vi "CalcData.vi"(8 "error in (no error)":errorcluster, 10 "Complex Data (in)":csg[](array[numeric])) -> (0 "error out":errorcluster, 2 "Array out":csg[](array[numeric]))   [LabVIEW 2014]
uses:
  GlobalVariables.vi
  <vilib>/rvi/interface/RandomDataEmulation/nirviRandomDataDMAMethods.vi
  <vilib>/rvi/interface/nirviMethod/nirviMethod.xnode
  Fpga-Version/PXI-7953R/Fft.vi
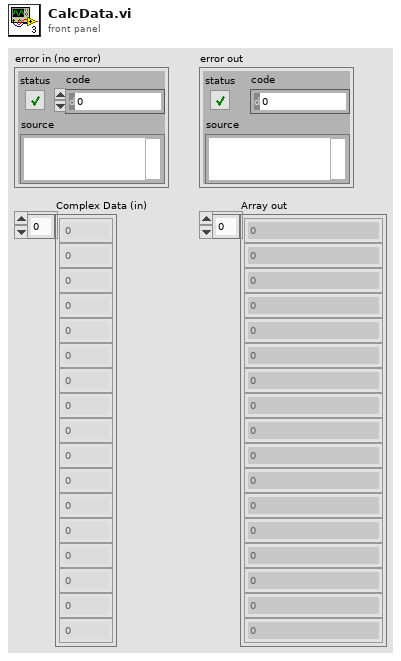
[diagram p1: front panel]
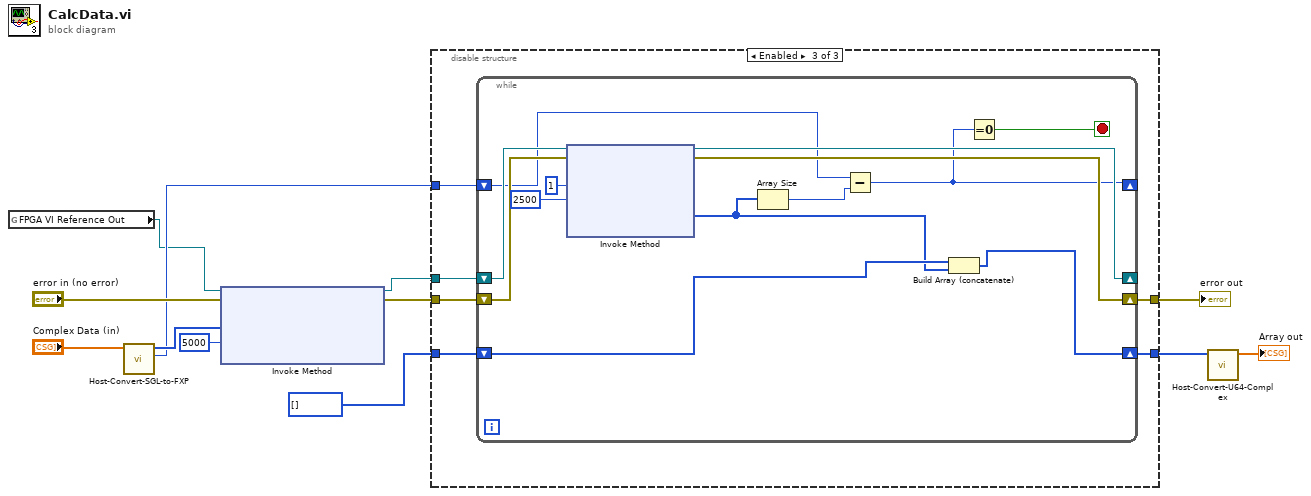
[diagram p0: block diagram]
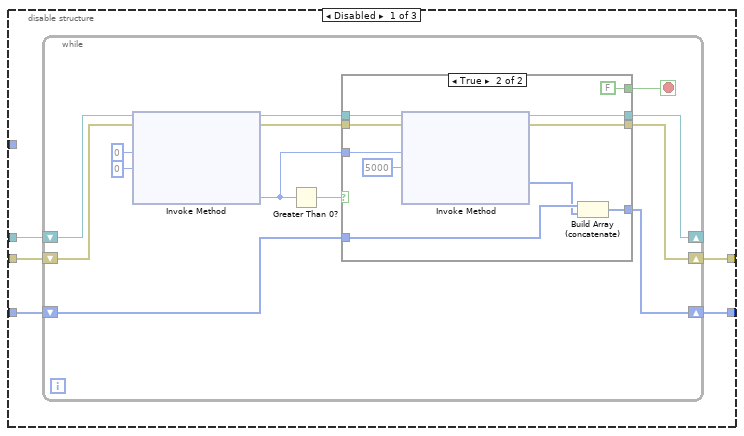
[diagram p2: hidden frame]
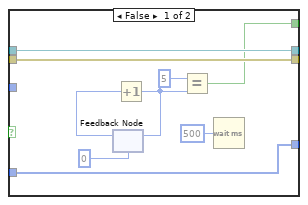
[diagram p3: hidden frame]
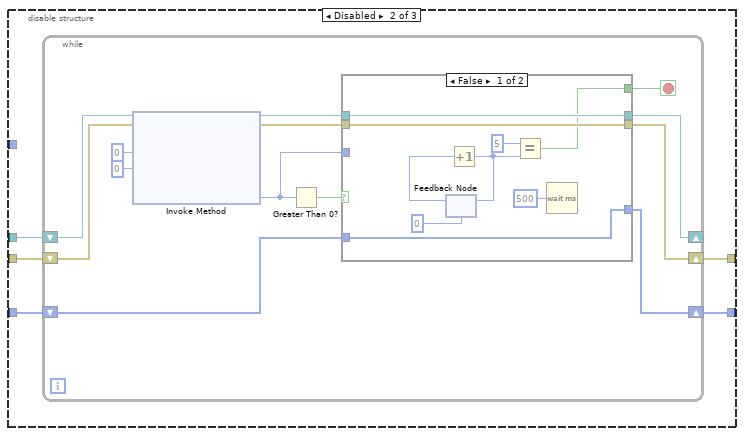
[diagram p4: hidden frame]
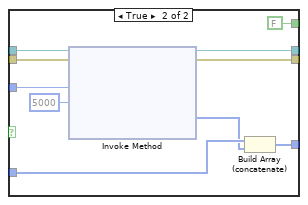
[diagram p5: hidden frame]
diagram:
  n1 = global read "GlobalVariables.vi" "FPGA VI Reference Out"() -> (w2:refnum<k20>)
  n2 = call "Host-Convert-SGL-to-FXP.vi"("Complex Data (in)"="Complex Data (in)") -> ("[FPGA] Array Size"=w3:u64, "Complex Data Ready for FPGA (out)"=w12:u64[])  [unwired: 9 in]
  n3 = xnode "Invoke Method"("FPGA VI Reference In"=w2, "error in"="error in (no error)", "Data"=w12, "Timeout (ms)"=5000) -> ("FPGA VI Reference Out"=w6:refnum<k20>, "error out"=w7:errorcluster)  [unwired: 1 out]
  n4 = disable-structure shown="Enabled" {
    disable-tunnel: [w17 w54 w88] -> w10
    disable-tunnel: u64[] [] -> [w16 w53 w90]
    disable-tunnel: [w15 w52 w89] -> w8
    disable-tunnel: w7 -> [w14 w51 w91]
    disable-tunnel: w6 -> [w13 w50 w92]
    disable-tunnel: w3 -> [_ _ w87]
    frame Disabled {
      n5 = while {
        shift-right: [w19] -> _
        shift-left: w13 -> [w30]
        shift-right: [w20] -> w15
        shift-left: w14 -> [w21]
        shift-right: [w24] -> w17
        shift-left: w16 -> [w23]
        stop <- w18 stop-if-true
        n6 = xnode "Invoke Method"("FPGA VI Reference In"=w30, "error in"=w21, "Number of Elements"=u32 0, "Timeout (ms)"=0) -> ("FPGA VI Reference Out"=w26:refnum<k20>, "error out"=w22:errorcluster, "Elements Remaining"=w25:u32)  [unwired: 1 out]
        n7 = Greater Than 0?(x=w25) -> (x > 0?=w27:bool)
        n8 = case shown="True" w27 {
          tunnel: w26 -> [w37 w49]
          tunnel: w25 -> [_ w48]
          tunnel: [w39 w44] -> w24
          tunnel: w23 -> [w39 w46]
          tunnel: w22 -> [w38 w43]
          tunnel: [w38 w42] -> w20
          tunnel: [w37 w41] -> w19
          tunnel: [w32 FALSE] -> w18
          frame False {
            n9 = feedback #1(0) -> (w35:i32)
            n10 = Increment(x=w35) -> (x+1=w34:i32)
            n11 = feedback-in #1(w34) -> ()
            n12 = Equal?(x=5, y=w34) -> (x = y?=w32:bool)
            n13 = Wait (ms)(milliseconds to wait=u32 500) -> ()  [unwired: 1 out]
          }
          frame True {
            n14 = xnode "Invoke Method"("FPGA VI Reference In"=w49, "error in"=w43, "Number of Elements"=w48, "Timeout (ms)"=5000) -> ("FPGA VI Reference Out"=w41:refnum<k20>, "error out"=w42:errorcluster, "Data"=w45:u64[])  [unwired: 1 out]
            n15 = Build Array (concatenate)(w46, w45) -> (w44:u64[])
          }
        }
      }
    }
    frame Disabled {
      n16 = while {
        shift-right: [w56] -> _
        shift-left: w50 -> [w67]
        shift-right: [w57] -> w52
        shift-left: w51 -> [w58]
        shift-right: [w61] -> w54
        shift-left: w53 -> [w60]
        stop <- w55 stop-if-true
        n17 = xnode "Invoke Method"("FPGA VI Reference In"=w67, "error in"=w58, "Number of Elements"=u32 0, "Timeout (ms)"=0) -> ("FPGA VI Reference Out"=w63:refnum<k20>, "error out"=w59:errorcluster, "Elements Remaining"=w62:u32)  [unwired: 1 out]
        n18 = Greater Than 0?(x=w62) -> (x > 0?=w64:bool)
        n19 = case shown="False" w64 {
          tunnel: w63 -> [w74 w86]
          tunnel: w62 -> [_ w85]
          tunnel: [w76 w81] -> w61
          tunnel: w60 -> [w76 w83]
          tunnel: w59 -> [w75 w80]
          tunnel: [w75 w79] -> w57
          tunnel: [w74 w78] -> w56
          tunnel: [w69 FALSE] -> w55
          frame False {
            n20 = feedback #2(0) -> (w72:i32)
            n21 = Increment(x=w72) -> (x+1=w71:i32)
            n22 = feedback-in #2(w71) -> ()
            n23 = Equal?(x=5, y=w71) -> (x = y?=w69:bool)
            n24 = Wait (ms)(milliseconds to wait=u32 500) -> ()  [unwired: 1 out]
          }
          frame True {
            n25 = xnode "Invoke Method"("FPGA VI Reference In"=w86, "error in"=w80, "Number of Elements"=w85, "Timeout (ms)"=5000) -> ("FPGA VI Reference Out"=w78:refnum<k20>, "error out"=w79:errorcluster, "Data"=w82:u64[])  [unwired: 1 out]
            n26 = Build Array (concatenate)(w83, w82) -> (w81:u64[])
          }
        }
      }
    }
    frame Enabled {
      n27 = while {
        shift-right: [w100] -> _
        shift-left: w92 -> [w105]
        shift-right: [w99] -> w89
        shift-left: w91 -> [w103]
        shift-right: [w101] -> w88
        shift-left: w90 -> [w102]
        shift-right: [w95] -> _
        shift-left: w87 -> [w97]
        stop <- w94 stop-if-true
        n28 = xnode "Invoke Method"("FPGA VI Reference In"=w105, "error in"=w103, "Number of Elements"=u32 1, "Timeout (ms)"=2500) -> ("FPGA VI Reference Out"=w100:refnum<k20>, "error out"=w99:errorcluster, "Data"=w98:u64[])  [unwired: 1 out]
        n29 = Array Size(array=w98) -> (size(s)=w96:i32)
        n30 = Subtract(x=w97, y=w96) -> (x-y=w95:u64)
        n31 = Build Array (concatenate)(w102, w98) -> (w101:u64[])
        n32 = Equal To 0?(x=w95) -> (x = 0?=w94:bool)
      }
    }
  }
  "error out" <- w8
  n33 = call "Host-Convert-U64-Complex.vi"("Array in"=w10) -> ("Array out"=→"Array out":csg[])  [unwired: 10 in]
